vi "GetDevList.vi"(6 "Legacy (f)?":bool, 8 "error in (no error)":errorcluster, 10 "CAL'd Only? (F = List All)":bool) -> (0 "error out":errorcluster, 1 "CAL Dates":string[](array[string]), 2 "DevNames":string[](array[string]), 3 "Serial Numbers":string[](array[string]), 5 "Module Types":T1[](array[typedef]))   [LabVIEW 2011]
uses:
  WebEngine/LIB/MODULES/Module_Types.ctl
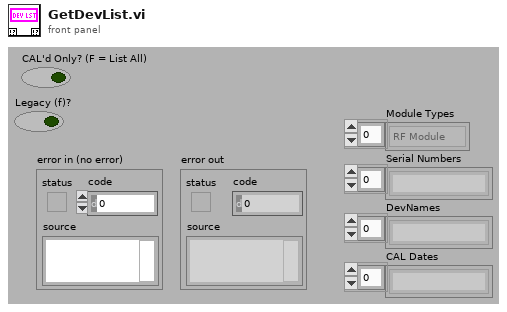
[diagram p1: front panel]
types:
  T1 = typedef "Module_Types.ctl" = enum16{"Unknown", "RF Module", "PA Module", "TR Module", "FE Module", "SW Module"}
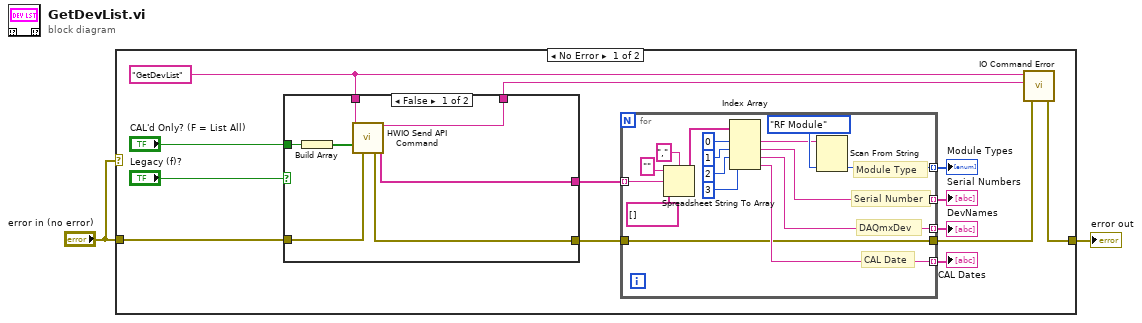
[diagram p0: block diagram]
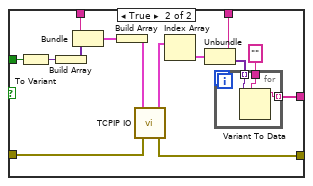
[diagram p2: hidden frame]
diagram:
  n1 = case shown="No Error" "error in (no error)" {
    tunnel: "error in (no error)" -> [w15 w56]
    tunnel: [w12 w56] -> w2
    frame No Error {
      w11 = "GetDevList"
      n2 = case shown="False" "Legacy (f)?" {
        tunnel: w15 -> [w19 w35]
        tunnel: [w18 w34] -> w14
        tunnel: w11 -> [w22 w33]
        tunnel: "CAL'd Only? (F = List All)" -> [w21 w29]
        tunnel: [w17 w24] -> w5
        tunnel: [w16 w23] -> w4
        frame False {
          n3 = Build Array(w21) -> (w20:bool[])
          n4 = call "HWIO Send API Command.vi"("Action"=w22, "Boolean"=w20, "error in (no error)"=w19) -> ("Action out"=w16:string, "error out"=w18:errorcluster, "String out"=w17:string[])  [unwired: 5 in, 5 out]
        }
        frame True {
          n5 = To Variant(anything=w29) -> (Variant=w28:variant)
          n6 = Build Array(w28) -> (w27:variant[])
          n7 = Bundle(w33, w27) -> (w36:cluster{string, variant[]})  [unwired: 1 out]
          n8 = Build Array(w36) -> (w30:cluster{string, variant[]}[])
          n9 = call "TCPIP IO.vi"("error in (no error)"=w35, "Commands"=w30) -> ("error out"=w34:errorcluster, "Responses"=w32:cluster{string, variant[]}[])  [unwired: 1 in, 3 out]
          n10 = Index Array(array=w32) -> (element=w31:cluster{string, variant[]})  [unwired: 1 in]
          n11 = Unbundle(w31) -> (w23:string, w25:variant[])
          n12 = for {
            tunnel: "" -> [w39]
            tunnel: w25 -> [w38] mode=indexing
            tunnel: [w37] -> w24 mode=indexing
            n13 = Variant To Data(type=w39, Variant=w38) -> (data=w37:string)  [unwired: 1 in, 1 out]
          }
        }
      }
      n14 = for {
        tunnel: [w41] -> w13
        tunnel: w14 -> [w41]
        tunnel: [w45] -> w9 mode=indexing
        tunnel: [w44] -> w8 mode=indexing
        tunnel: [w43] -> w7 mode=indexing
        tunnel: [w42] -> w6 mode=indexing
        tunnel: w5 -> [w40] mode=indexing
        # "CAL Date"
        # "DAQmxDev"
        # "Serial Number"
        # "Module Type"
        n15 = Spreadsheet String To Array(delimiter (Tab)=",", format string="", spreadsheet string=w40, array type (2D Dbl)=string[] []) -> (array=w50:string[])
        n16 = Index Array(array=w50, index #1=0 ("index"), index #2=1 ("index"), index #3=2 ("index"), index #4=3 ("index")) -> (element #1=w46:string, element #2=w44:string, element #3=w43:string, element #4=w42:string)
        n17 = Scan From String(input string=w46, default 1=Module_Types."RF Module" ("Module Type")) -> (output 1=w45:T1)  [unwired: 3 in, 3 out]
      }
      "Module Types" <- w9
      "Serial Numbers" <- w8
      "DevNames" <- w7
      "CAL Dates" <- w6
      n18 = call "IO Command Error.vi"("error in (no error)"=w13, "Command Returned (\"\")"=w4, "Command Sent (\"\")"=w11) -> ("error out"=w12:errorcluster)  [unwired: 4 out]
    }
    frame Error {
    }
  }
  "error out" <- w2
